vi "Inclinometer Output Max Range.vi"(11 "Data In":T1) -> (3 "Data Out":T1)   [LabVIEW 2018]
doc: "Assert Component\nAssert Name: Inclinometer Output Max Range\nData Type: Double Float\nDeveloped by Delacor\nEvaluation String: X < 4.500000\nDescription:"
uses:
  Users/Delacor/Documents/LabVIEW Data/Assert API Support/Templates/NC Templates/dbl.ctl
  <vilib>/Assert API/Core/Assert API Components/Failure Actions.ctl
  <vilib>/Assert API/Core/Assert API Components/Assert API Components.lvlib
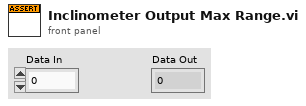
[diagram p1: front panel]
types:
  T1 = typedef "dbl.ctl" = dbl
  T2 = typedef "Assert API Components.lvlib/Failure Actions.ctl" = enum16{"None", "Log To File", "Pause Execution", "Abort Execution"}
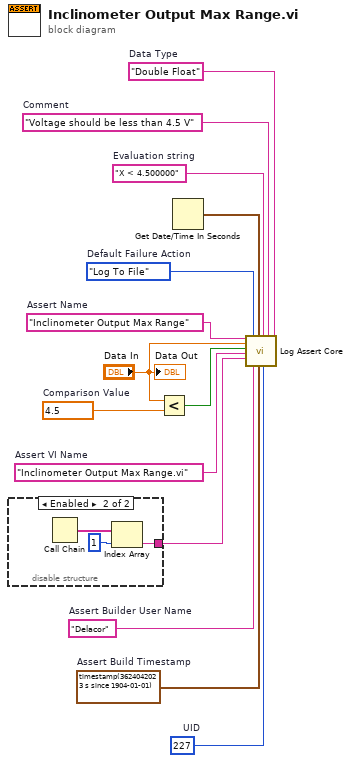
[diagram p0: block diagram]
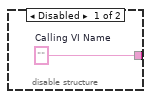
[diagram p2: hidden frame]
diagram:
  w2 = 227  # UID
  w4 = "Inclinometer Output Max Range.vi"  # Assert VI Name
  w5 = "Double Float"  # Data Type
  w6 = "Delacor"  # Assert Builder User Name
  w7 = timestamp(3624042023.5172305 s since 1904-01-01)  # Assert Build Timestamp
  w11 = "Voltage should be less than 4.5 V"  # Comment
  w8 = "X < 4.500000"  # Evaluation string
  w13 = Failure_Actions."Log To File"  # Default Failure Action
  w14 = "Inclinometer Output Max Range"  # Assert Name
  w12 = T1 4.5  # Comparison Value
  n1 = disable-structure shown="Enabled" {
    disable-tunnel: [w15 w16] -> w1
    frame Disabled {
      w15 = ""  # Calling VI Name
    }
    frame Enabled {
      n2 = Call Chain() -> (call chain=w17:string[])
      n3 = Index Array(array=w17, index=1) -> (element=w16:string)
    }
  }
  n4 = Less?(x="Data In", y=w12) -> (x < y?=w9:bool)
  n5 = Get Date/Time In Seconds() -> (seconds since 1Jan1904=w3:timestamp)
  n6 = call <vilib>:"Log Assert Core.vi"("Assert Name"=w14, "Data Value"="Data In", "Status"=w9, "Assert VI Name"=w4, "Calling VI Name"=w1, "Failure Action"=w13, "Assert Builder User Name"=w6, "Last Update"=w3, "Assert Build Timestamp"=w7, "Evaluation String"=w8, "Assert VI UID"=w2, "Comment"=w11, "Data Type"=w5) -> ()  [unwired: 7 in]
  "Data Out" <- "Data In"
